vi "Write Voltage.vi"(8 "error in":errorcluster, 10 "Voltage":dbl, 11 "57XX in":refnum<class "57XX.lvclass">) -> (0 "error out":errorcluster, 3 "57XX out":refnum<class "57XX.lvclass">)   [LabVIEW 2019, in "57XX.lvlib" / "57XX.lvclass"]
uses:
  Library/57XX.lvclass
  builds/Instruments/PowerSupply.lvlibp/Library/PowerSupply.lvclass
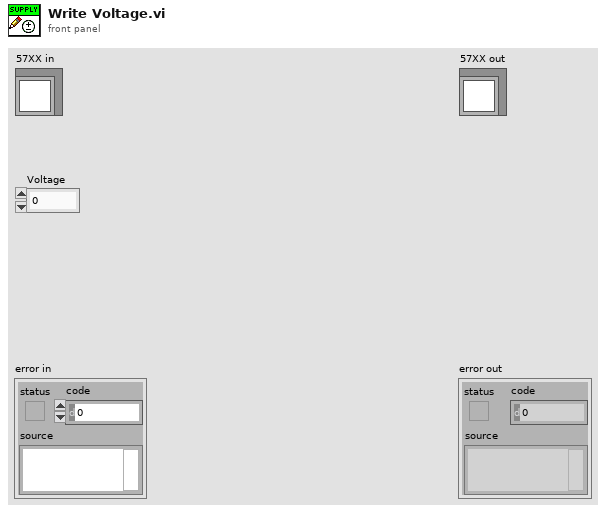
[diagram p1: front panel]
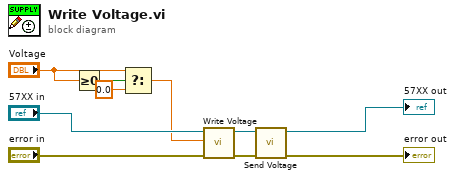
[diagram p0: block diagram]
diagram:
  n1 = Greater Or Equal To 0?(x="Voltage") -> (x >= 0?=w4:bool)
  n2 = Select(t="Voltage", s=w4, f=0.0) -> (s? t:f=w1:dbl)
  n3 = call-parent "Write Voltage.vi"("error in"="error in", "Voltage"=w1, "PowerSupply in"="57XX in") -> ("error out"=w5:errorcluster, "PowerSupply out"=w6:refnum<class "57XX.lvclass">)  [unwired: 7 in]
  n4 = call "Send Voltage.vi"("error in (no error)"=w5, "57XX in"=w6) -> ("error out"=→"error out":errorcluster, "57XX out"=→"57XX out":refnum<class "57XX.lvclass">)  [unwired: 8 in]
